vi "Ramp H out Cal.vi"(4 "Speed_Ref_Cal_H":dbl, 5 "Numeric":dbl, 6 "Speed \nReferance H":dbl, 7 "Engine Speed/Torque H":bool, 8 "H":dbl[](array[numeric]), 9 "Ramp H Active":bool, 10 "Output Ramp H in":dbl, 11 "Direction H":bool) -> (3 "Output Ramp H out":dbl)   [LabVIEW 2018]
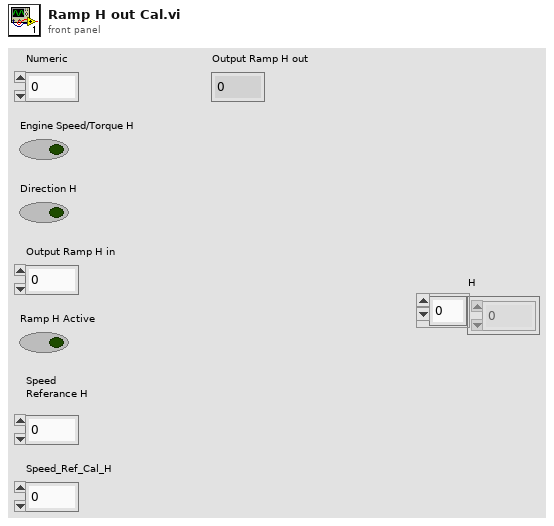
[diagram p1: front panel]
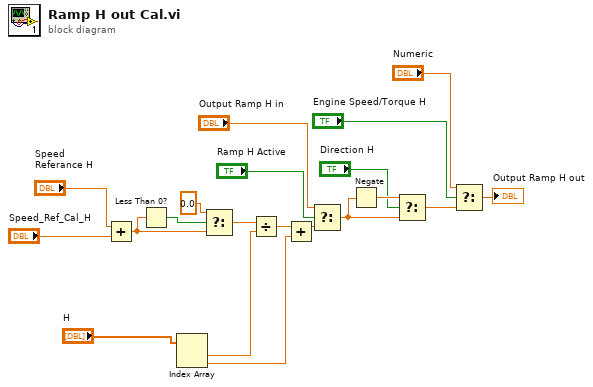
[diagram p0: block diagram]
diagram:
  n1 = Add(x="Speed \nReferance H", y="Speed_Ref_Cal_H") -> (x+y=w17:dbl)
  n2 = Less Than 0?(x=w17) -> (x < 0?=w5:bool)
  n3 = Index Array(array="H") -> (element #1=w3:dbl, element #2=w1:dbl)  [unwired: 2 in]
  n4 = Select(t=0.0, s=w5, f=w17) -> (s? t:f=w7:dbl)
  n5 = Divide(x=w7, y=w3) -> (x/y=w18:dbl)
  n6 = Add(x=w18, y=w1) -> (x+y=w2:dbl)
  n7 = Select(t="Output Ramp H in", s="Ramp H Active", f=w2) -> (s? t:f=w19:dbl)
  n8 = Negate(x=w19) -> (-x=w9:dbl)
  n9 = Select(t=w9, s="Direction H", f=w19) -> (s? t:f=w20:dbl)
  n10 = Select(t="Numeric", s="Engine Speed/Torque H", f=w20) -> (s? t:f=→"Output Ramp H out":dbl)
